vi "PAN_TCPSERVER_Server.vi"(3 "open panel":bool, 4 "log":bool, 5 "logfile":path, 6 "max instances":i8=10, 7 "callerID":string, 9 "notifier In":refnum<notifier>, 10 "messages from sock":refnum<queue>, 11 "listener ID":refnum<k5>) -> ()   [LabVIEW 2016]
uses:
  private/vis/PAN_TCPSERVER_MsgStruct.ctl
panel:
  out "last error":errorcluster
  in  "caller path":path
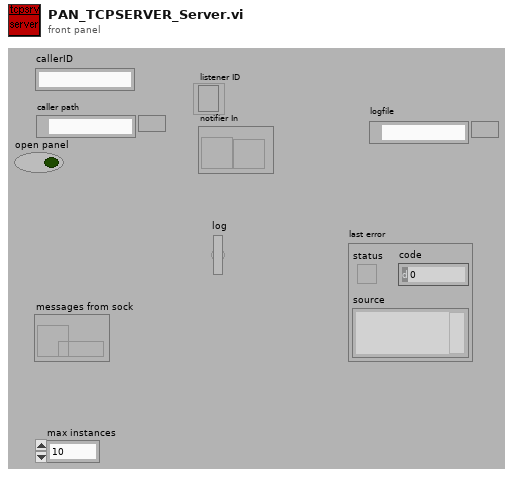
[diagram p1: front panel]
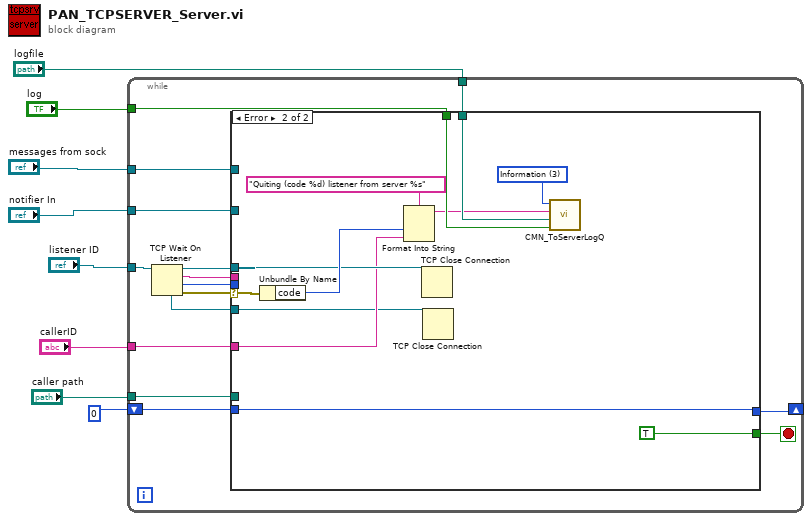
[diagram p0: block diagram]
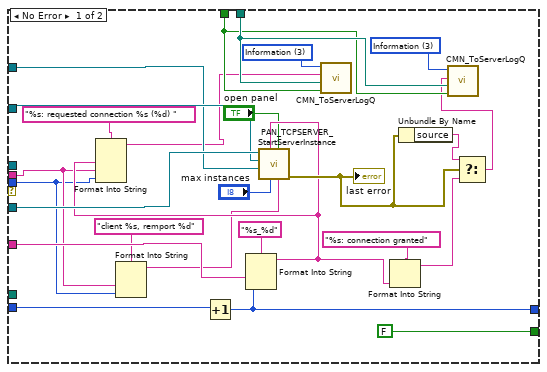
[diagram p2: hidden frame]
diagram:
  n1 = while {
    tunnel: "listener ID" -> [w23]
    tunnel: "notifier In" -> [w20]
    tunnel: "messages from sock" -> [w19]
    tunnel: "callerID" -> [w18]
    tunnel: "caller path" -> [w17]
    shift-right: [w14] -> _
    shift-left: 0 -> [w15]
    tunnel: "logfile" -> [w12]
    tunnel: "log" -> [w11]
    stop <- w16 stop-if-true
    n2 = TCP Wait On Listener(11:w23) -> (0:w22:errorcluster, 1:w9:u16, 2:w10:string, 3:w13:refnum<k5>, 4:w21:refnum<k5>)  [unwired: 1 in, 2 out]
    n3 = case shown="Error" w22 {
      selector: w22 -> [_ w54]
      tunnel: w21 -> [w49 w50]
      tunnel: w20 -> [w48 _]
      tunnel: w19 -> [w47 _]
      tunnel: w18 -> [w32 w51]
      tunnel: w17 -> [_ _]
      tunnel: [FALSE TRUE] -> w16
      tunnel: w15 -> [w45 w60]
      tunnel: [w43 w60] -> w14
      tunnel: w13 -> [_ w52]
      tunnel: w12 -> [w39 w58]
      tunnel: w11 -> [w38 w57]
      tunnel: w10 -> [w26 _]
      tunnel: w9 -> [w25 _]
      frame No Error {
        w40 = u16 3 items=["command", "imediateReply", "Callback Reply", "Information", "none"] ("type")
        w41 = u16 3 items=["command", "imediateReply", "Callback Reply", "Information", "none"] ("type")
        n4 = Format Into String(format string="client %s, remport %d", w26, w25) -> (resulting string=w24:string)  [unwired: 2 in, 1 out]
        n5 = Increment(x=w45) -> (x+1=w43:i32)
        n6 = Format Into String(format string="%s_%d", w32, w43) -> (resulting string=w30:string)  [unwired: 2 in, 1 out]
        n7 = Format Into String(format string="%s: requested connection %s (%d) " ("string"), w30, w26, w25) -> (resulting string=w36:string)  [unwired: 2 in, 1 out]
        n8 = call "PAN_TCPSERVER_StartServerInstance.vi"("client params"=w24, "open panel"="open panel", "max instances"="max instances", "ID"=w30, "messages from sock Q"=w47, "notifier In"=w48, "sock ID"=w49) -> ("error out"=w35:errorcluster)  [unwired: 1 in, 3 out]
        "last error" <- w35
        n9 = call "CMN_ToServerLogQ.vi"("Log"=w38, "file"=w39, "string"=w36, "type"=w41) -> ()  [unwired: 2 in, 5 out]
        n10 = Format Into String(format string="%s: connection granted" ("f"), w30) -> (resulting string=w29:string)  [unwired: 2 in, 1 out]
        n11 = Unbundle By Name(w35) -> ("source"=w34:string)
        n12 = Select(t=w34, s=w35, f=w29) -> (s? t:f=w33:string)
        n13 = call "CMN_ToServerLogQ.vi"("Log"=w38, "file"=w39, "string"=w33, "type"=w40) -> ()  [unwired: 2 in, 5 out]
      }
      frame Error {
        w59 = u16 3 items=["command", "imediateReply", "Callback Reply", "Information", "none"] ("type")
        (unwired) TRUE
        n14 = Unbundle By Name(w54) -> ("code"=w53:i32)
        n15 = Format Into String(format string="Quiting (code %d) listener from server %s", w53, w51) -> (resulting string=w55:string)  [unwired: 2 in, 1 out]
        n16 = TCP Close Connection(connection ID=w52) -> ()  [unwired: 1 in, 3 out]
        n17 = TCP Close Connection(connection ID=w50) -> ()  [unwired: 1 in, 3 out]
        n18 = call "CMN_ToServerLogQ.vi"("Log"=w57, "file"=w58, "string"=w55, "type"=w59) -> ()  [unwired: 2 in, 5 out]
      }
    }
  }
